vi "VSS Detection Frame.vi"(4 "time stamp":timestamp, 8 "error in":errorcluster, 9 "Array":u8[](array[numeric]) format="%02x") -> (0 "error out":errorcluster, 1 "array w/ subset deleted out":u8[](array[numeric]), 3 "Detection Frame":T1 {"robots_blue"."height" format="%+4.3f"; "robots_blue"."pixel_y" format="%+4.3f"; "robots_blue"."pixel_x" format="%+4.3f"; "robots_blue"."orientation" format="%+4.3f"; "robots_blue"."y" format="%+4.3f"; "robots_blue"."confidence" format="%4.3f"; "robots_blue"."x" format="%+4.3f"; "robots_yellow"."height" format="%+4.3f"; "robots_yellow"."pixel_y" format="%+4.3f"; "robots_yellow"."pixel_x" format="%+4.3f"; "robots_yellow"."orientation" format="%+4.3f"; "robots_yellow"."y" format="%+4.3f"; "robots_yellow"."confidence" format="%4.3f"; "robots_yellow"."x" format="%+4.3f"})   [LabVIEW 2018]
uses:
  SSL Detection Frame.ctl
  SSL Detection Robot.ctl
  <vilib>/Analysis/Matrix/Datatypes/RealMatrix.ctl
  SSL Detection Ball.ctl
  <vilib>/Analysis/Matrix/NI_Matrix.lvlib
panel:
  out "size(s) 3":i32
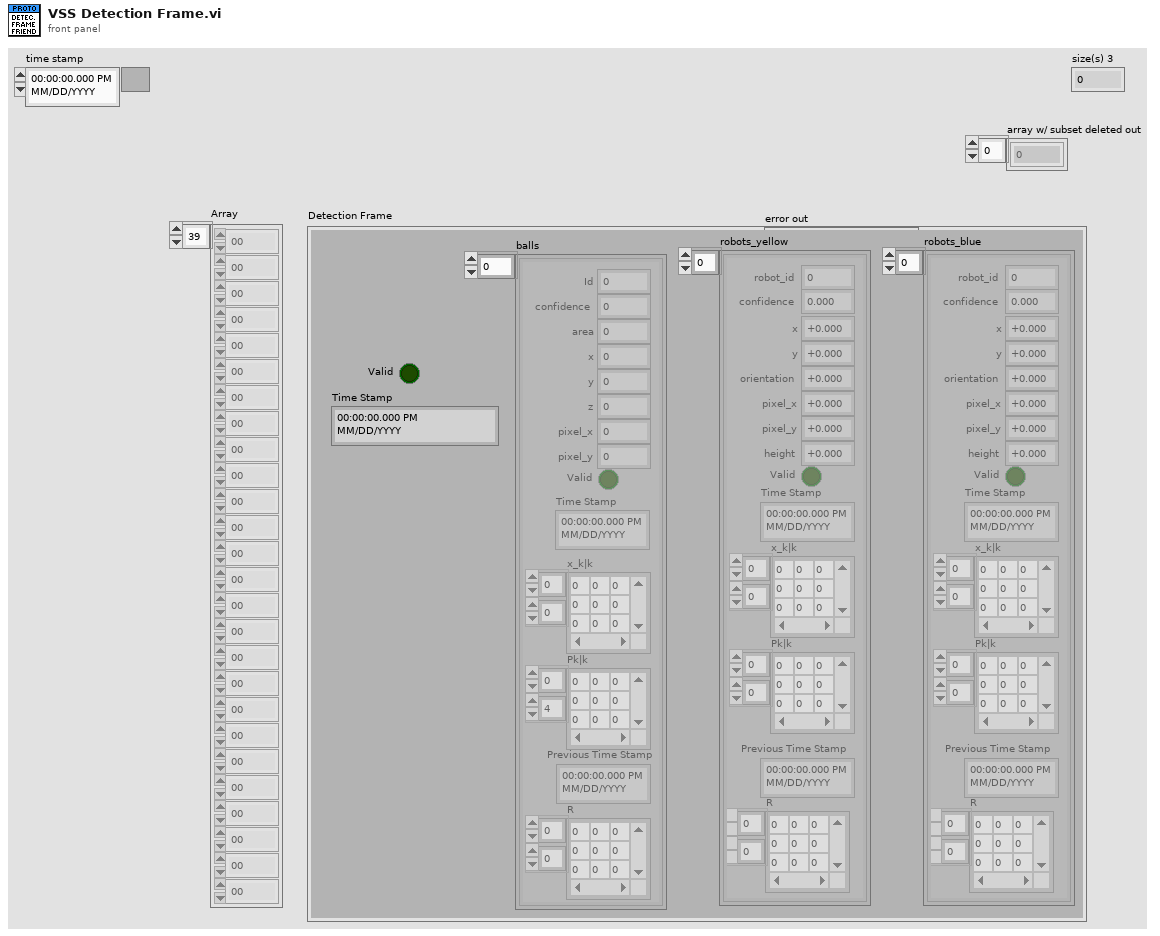
[diagram p1: front panel]
types:
  T1 = typedef "SSL Detection Frame.ctl" = cluster{"robots_yellow":T2[], "robots_blue":T2[], "balls":T4[], "Valid":bool, "Time Stamp":timestamp}
  T2 = typedef "SSL Detection Robot.ctl" = cluster{"x":sgl, "robot_id":u32, "confidence":sgl, "y":sgl, "orientation":sgl, "pixel_x":sgl, "pixel_y":sgl, "height":sgl, "Valid":bool, "Time Stamp":timestamp, "x_k|k":T3, "Pk|k":T3, "Previous Time Stamp":timestamp, "R":T3}
  T3 = typedef "NI_Matrix.lvlib/RealMatrix.ctl" = dbl[][]
  T4 = typedef "SSL Detection Ball.ctl" = cluster{"x":sgl, "area":u32, "confidence":sgl, "y":sgl, "z":sgl, "pixel_x":sgl, "pixel_y":sgl, "Valid":bool, "Time Stamp":timestamp, "x_k|k":T3, "Pk|k":T3, "Id":u32, "Previous Time Stamp":timestamp, "R":T3}
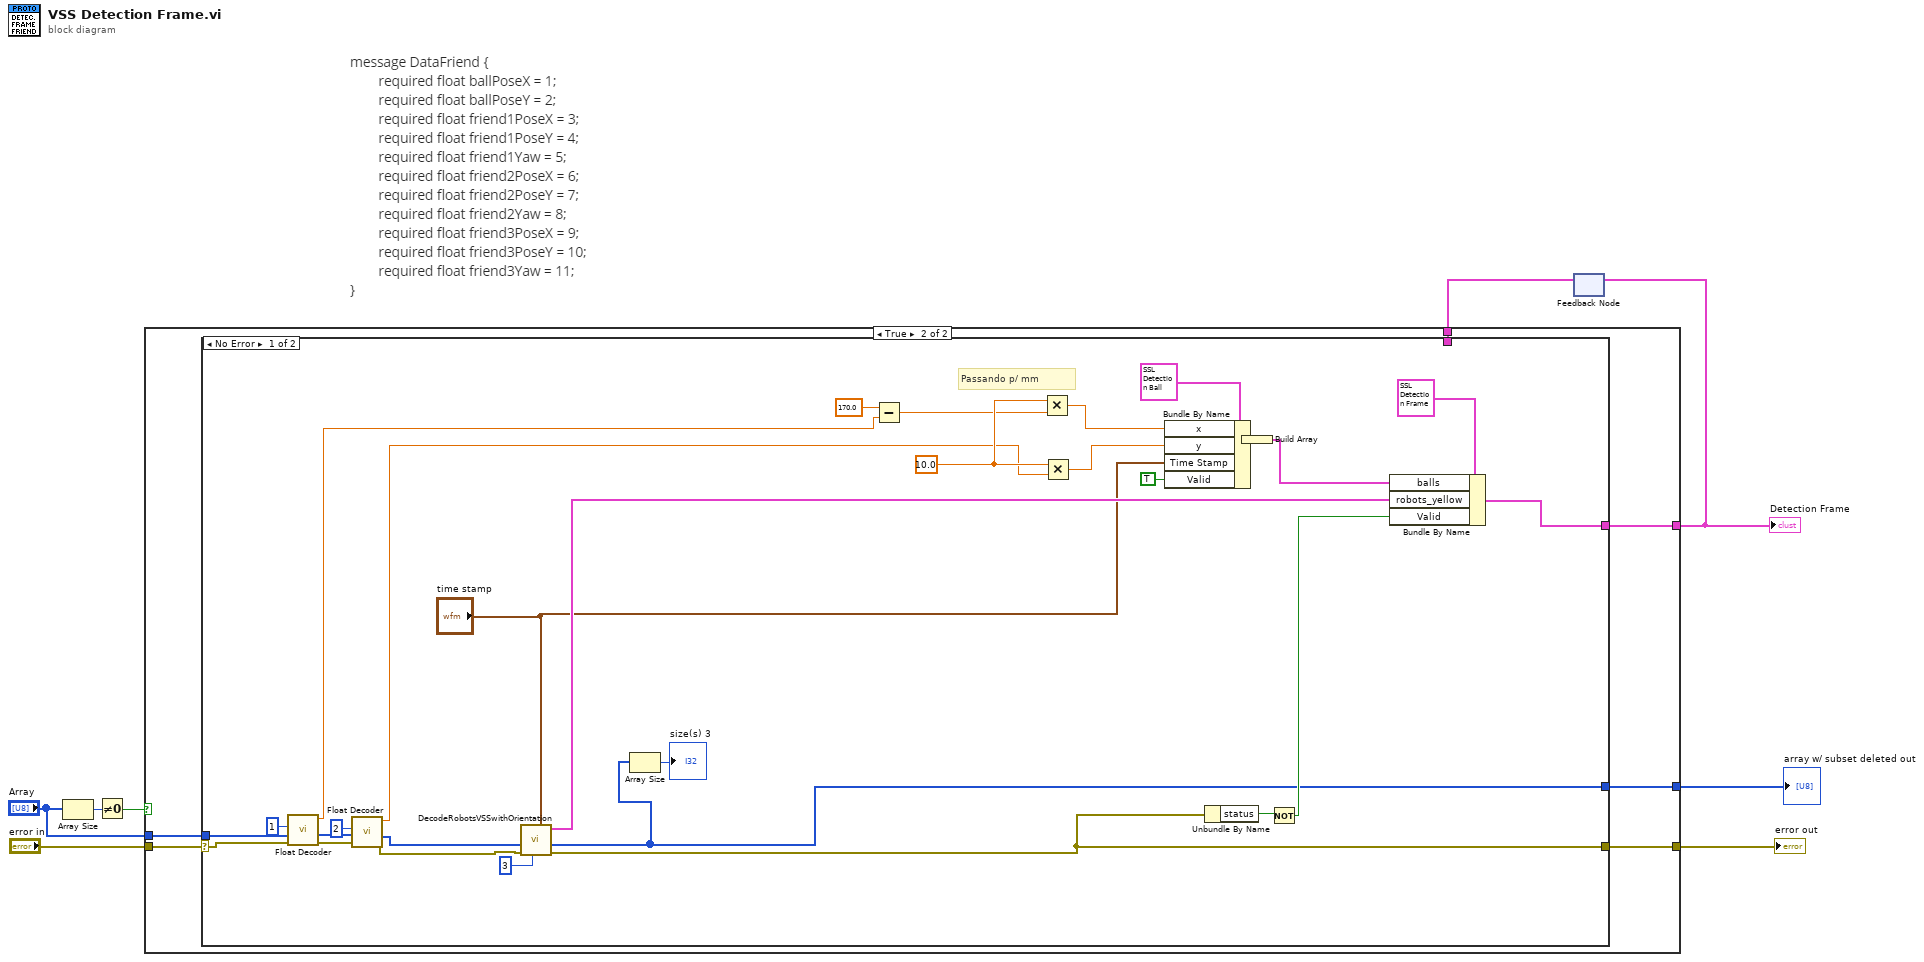
[diagram p0: block diagram]
diagram:
  n1 = Array Size(array="Array") -> (size(s)=w6:i32)
  n2 = Not Equal To 0?(x=w6) -> (x != 0?=w4:bool)
  n3 = feedback #1() -> (w3:T1)  [unwired: 1 in]
  n4 = case shown="True" w4 {
    tunnel: "error in" -> [_ w16]
    tunnel: "Array" -> [w9 w15]
    tunnel: [_ w14] -> w5
    tunnel: [w10 w13] -> w2
    tunnel: w3 -> [w10 w12]
    tunnel: [w9 w11] -> w1
    frame False {
    }
    frame True {
      n5 = case shown="No Error" w16 {
        selector: w16 -> [w36 w48]
        tunnel: [w40 w48] -> w14
        tunnel: w15 -> [w37 w46]
        tunnel: [w43 w47] -> w13
        tunnel: w12 -> [_ w47]
        tunnel: [w28 w46] -> w11
        frame No Error {
          w25 = 10.0 ("x")
          # "Passando p/ mm"
          n6 = call "Float Decoder.vi"("error in (no error)"=w36, "Array"=w37, "Key"=1) -> ("error out"=w35:errorcluster, "array w/ subset deleted"=w34:u8[], "Float"=w18:sgl)  [unwired: 5 in, 1 out]
          n7 = call "Float Decoder.vi"("error in (no error)"=w35, "Array"=w34, "Key"=2) -> ("error out"=w32:errorcluster, "array w/ subset deleted"=w33:u8[], "Float"=w23:sgl)  [unwired: 5 in, 1 out]
          n8 = call "DecodeRobotsVSSwithOrientation.vi"("time stamp"="time stamp", "offset"=3, "error in (no error)"=w32, "array w/ subset deleted in"=w33) -> ("error out"=w40:errorcluster, "array w/ subset deleted out"=w28:u8[], "Array"=w42:T2[])  [unwired: 4 in]
          n9 = Array Size(array=w28) -> (size(s)=→"size(s) 3":i32)
          n10 = Subtract(x=170.0, y=w18) -> (x-y=w17:dbl)
          n11 = Multiply(x=w25, y=w17) -> (x*y=w24:dbl)
          n12 = Multiply(x=w25, y=w23) -> (x*y=w20:dbl)
          n13 = Bundle By Name(cluster=T4 {"x"=0.0, "area"=0, "confidence"=0.0, "y"=0.0, "z"=0.0, "pixel_x"=0.0, "pixel_y"=0.0, "Valid"=FALSE, "Time Stamp"=timestamp(0 s since 1904-01-01), "x_k|k"=[], "Pk|k"=[], "Id"=0, "Previous Time Stamp"=timestamp(0 s since 1904-01-01), "R"=[]} ("element"), "x"=w24, "y"=w20, "Time Stamp"="time stamp", "Valid"=TRUE) -> (w29:T4)
          n14 = Unbundle By Name(w40) -> ("status"=w41:bool)
          n15 = Build Array(w29) -> (w26:T4[])
          n16 = Not(x=w41) -> (.not. x?=w44:bool)
          n17 = Bundle By Name(cluster=T1 {"robots_yellow"=[], "robots_blue"=[], "balls"=[], "Valid"=FALSE, "Time Stamp"=timestamp(0 s since 1904-01-01)} ("Detection Frame 2"), "balls"=w26, "robots_yellow"=w42, "Valid"=w44) -> (w43:T1)
        }
        frame Error {
        }
      }
    }
  }
  "error out" <- w5
  "Detection Frame" <- w2
  "array w/ subset deleted out" <- w1
  n18 = feedback-in #1(w2) -> ()
